vi "Write Digital Output State.vi"(8 "error in (no error)":errorcluster, 9 "Digital Output State":bool, 10 "Digital Output Selection":i32, 11 "DigitalIO in":refnum<class "DigitalIO.lvclass">) -> (0 "error out":errorcluster, 3 "DigitalIO out":refnum<class "DigitalIO.lvclass">)   [LabVIEW 2018, in "DigitalIO.lvlib" / "DigitalIO.lvclass"]
uses:
  DigitalIO.lvclass
  DigitalIO.lvclass/DigitalIO.ctl
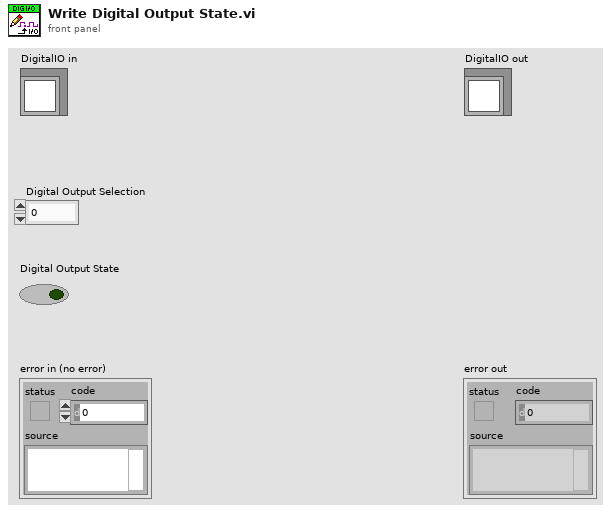
[diagram p1: front panel]
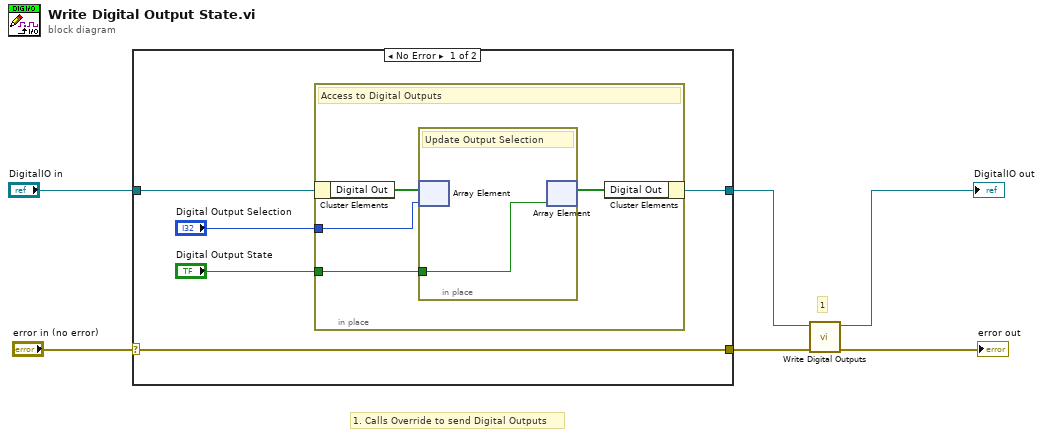
[diagram p0: block diagram]
diagram:
  # "1. Calls Override to send Digital Outputs"
  # "1"
  n1 = case shown="No Error" "error in (no error)" {
    selector: "error in (no error)" -> [w11 w18]
    tunnel: [w11 w18] -> w3
    tunnel: [w7 w17] -> w4
    tunnel: "DigitalIO in" -> [w10 w17]
    frame No Error {
      n2 = in-place {
        in-place-border: "Digital Output Selection" -> [w14]
        in-place-border: "Digital Output State" -> [w13]
        # "Access to Digital Outputs"
        n3 = in-place-cluster #1(w10) -> ("Digital Out"=w15:bool[])
        n4 = in-place {
          in-place-border: w13 -> [w16]
          # "Update Output Selection"
          n5 = in-place-array #2(w15, w14) -> ()  [unwired: 1 out]
          n6 = in-place-array #2(w16) -> (w12:bool[])  [unwired: 1 out]
        }
        n7 = in-place-cluster #1("Digital Out"=w12) -> (w7:refnum<class "DigitalIO.lvclass">)
      }
    }
    frame Error {
    }
  }
  n8 = call-dynamic "Write Digital Outputs.vi"("error in (no error)"=w3, "DigitalIO in"=w4) -> ("error out"=→"error out":errorcluster, "DigitalIO out"=→"DigitalIO out":refnum<class "DigitalIO.lvclass">)  [unwired: 8 in]
